vi "Obtain Broadcast Events.vi"(8 "error in (no error)":errorcluster, 10 "Create New?":bool) -> (0 "error out":errorcluster, 2 "FlexiFlowInterfaceCH2 Broadcast Events":T1)   [LabVIEW 2024, in "FlexiFlowInterfaceCH2.lvlib"]
doc: "This VI Obtains/Creates the Broadcast events that will be used for other modules to register to receive messages from the module that owns this VI.\n\n<b>NOTE</b>: The contents of this VI are automatically generated and modified by the <b>Tools > Delacor > DQMH</b> utilities. Consider using those utilities instead of making your own modifications to this VI.\n_____\nBased on Delacor QMH Project Template 3.1.0.34."
uses:
  FlexiFlowInterfaceCH2.lvlib
  Broadcast Events--cluster.ctl
  Did Init Argument--cluster.ctl
  Status Updated Argument--cluster.ctl
  Error Reported Argument--cluster.ctl
  Stop Argument--cluster.ctl
  Get Module Execution Status Argument--cluster.ctl
  Broadcast Device States Argument--cluster.ctl
  Modbus Flexi-Flow State--cluster.ctl
  <vilib>/Plasmionique/MB Master/MB_Master_TCP/MB_Master_TCP.lvclass
  Device Type--enum.ctl
  Modbus Flexi-Flow Controls--cluster.ctl
  Modbus Flexi-Flow API/Control Mode--enum.ctl
  Modbus Flexi-Flow API/Control Function Values--enum.ctl
  Modbus Flexi-Flow Measure State--cluster.ctl
  Broadcast State (Data Map) Argument--cluster.ctl
  Modbus Flexi-Flow API/Bronkhorst Flexi-Flow ModbusTCP API.lvlib
panel:
  # "NOTE: The contents of this VI are automatically generated and modified by the Tools > Delacor > DQMH utilities. Consider using those utilities instead of making your own modifications to this VI."
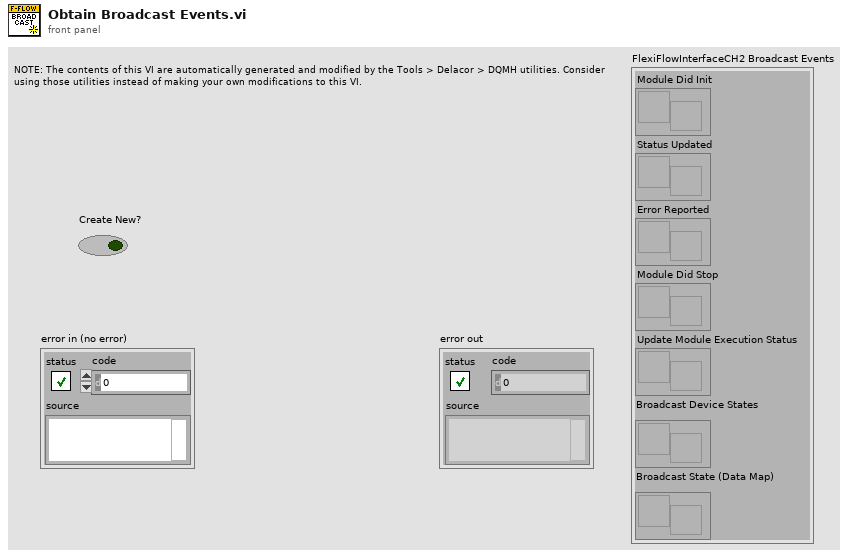
[diagram p1: front panel]
types:
  T1 = typedef "FlexiFlowInterfaceCH2.lvlib/Broadcast Events--cluster.ctl" = cluster{"Module Did Init":refnum<user-event>, "Status Updated":refnum<user-event>, "Error Reported":refnum<user-event>, "Module Did Stop":refnum<user-event>, "Update Module Execution Status":refnum<user-event>, "Broadcast Device States":refnum<user-event>, "Broadcast State (Data Map)":refnum<user-event>}
  T2 = typedef "FlexiFlowInterfaceCH2.lvlib/Broadcast State (Data Map) Argument--cluster.ctl" = cluster{"Data Table":map{string, dbl}}
  T3 = typedef "FlexiFlowInterfaceCH2.lvlib/Broadcast Device States Argument--cluster.ctl" = cluster{"Flexi-Flow Devices":T4[]}
  T4 = typedef "FlexiFlowInterfaceCH2.lvlib/Modbus Flexi-Flow State--cluster.ctl" = cluster{"Type":T5, "Label":string, "User Tag":string, "MB_TCP session":refnum<class "MB_Master_TCP.lvclass">, "Control State":T6, "Measurement State":T9}
  T5 = typedef "FlexiFlowInterfaceCH2.lvlib/Device Type--enum.ctl" = enum16{"Mass Flow Controller", "Mass Flow Meter"}
  T6 = typedef "FlexiFlowInterfaceCH2.lvlib/Modbus Flexi-Flow Controls--cluster.ctl" = cluster{"Control Mode":T7, "Function":T8, "FSetpoint":sgl, "Flow Capacity Unit":string, "Setpoint Slope":u16, "P1Setpoint":sgl, "P2Setpoint":sgl}
  T7 = typedef "Bronkhorst Flexi-Flow ModbusTCP API.lvlib/Control Mode--enum.ctl" = u16
  T8 = typedef "Bronkhorst Flexi-Flow ModbusTCP API.lvlib/Control Function Values--enum.ctl" = enum16{"Flow", "Upstream pressure", "Downstream pressure", "Flow with upstream pressure limit", "Flow with downstream pressure limit", "Upstream pressure with flow limit", "Downstream pressure with flow limit"}
  T9 = typedef "FlexiFlowInterfaceCH2.lvlib/Modbus Flexi-Flow Measure State--cluster.ctl" = cluster{"Fmeasure":dbl, "P1measure":sgl, "P2measure":sgl}
  T10 = typedef "FlexiFlowInterfaceCH2.lvlib/Get Module Execution Status Argument--cluster.ctl" = cluster{"Running?":bool}
  T11 = typedef "FlexiFlowInterfaceCH2.lvlib/Stop Argument--cluster.ctl" = cluster{"Origin":string, "Exit via Stop Module Req?":bool, "Wait for Module to stop?":bool}
  T12 = typedef "FlexiFlowInterfaceCH2.lvlib/Error Reported Argument--cluster.ctl" = cluster{"Error":errorcluster, "Additional Information":string, "Module Name":string}
  T13 = typedef "FlexiFlowInterfaceCH2.lvlib/Status Updated Argument--cluster.ctl" = cluster{"Status":string}
  T14 = typedef "FlexiFlowInterfaceCH2.lvlib/Did Init Argument--cluster.ctl" = cluster{"Init?":bool, "Info":string}
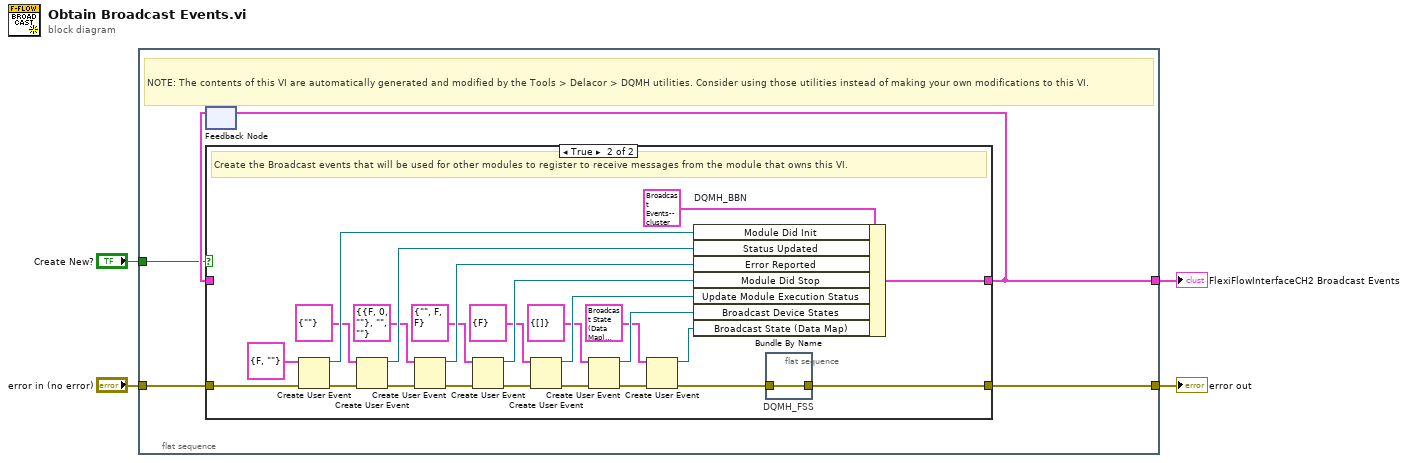
[diagram p0: block diagram]
diagram:
  n1 = flat-sequence {
    tunnel: [w9] -> w4
    tunnel: "error in (no error)" -> [w8]
    tunnel: [w6] -> w2
    tunnel: "Create New?" -> [w5]
    frame #0 {
      # "NOTE: The contents of this VI are automatically generated and modified by the Tools > Delacor > DQMH utilities. Consider using those utilities instead of making your own modifications to this VI."
      n2 = feedback #1() -> (w7:T1)  [unwired: 1 in]
      n3 = case shown="True" w5 {
        tunnel: [w10 w21] -> w9
        tunnel: w8 -> [w10 w36]
        tunnel: [w11 w33] -> w6
        tunnel: w7 -> [w11 _]
        frame False {
          # "Obtain the Broadcast events that were created in a previous call to this VI."
        }
        frame True {
          # "Create the Broadcast events that will be used for other modules to register to receive messages from the module that owns this VI."
          n4 = Create User Event(user event datatype=T14 {"Init?"=FALSE, "Info"=""} ("Did Init Argument"), error in=w36) -> (user event=w34:refnum<user-event>, error out=w31:errorcluster)
          n5 = Create User Event(user event datatype=T13 {"Status"=""} ("Status Updated Argument"), error in=w31) -> (user event=w28:refnum<user-event>, error out=w30:errorcluster)
          n6 = Create User Event(user event datatype=T12 {"Error"={"status"=FALSE, "code"=0, "source"=""}, "Additional Information"="", "Module Name"=""} ("Error Reported Argument"), error in=w30) -> (user event=w25:refnum<user-event>, error out=w27:errorcluster)
          n7 = Create User Event(user event datatype=T11 {"Origin"="", "Exit via Stop Module Req?"=FALSE, "Wait for Module to stop?"=FALSE} ("Stop Argument"), error in=w27) -> (user event=w23:refnum<user-event>, error out=w22:errorcluster)
          n8 = Create User Event(user event datatype=T10 {"Running?"=FALSE} ("Get Module Execution Status Argument"), error in=w22) -> (user event=w19:refnum<user-event>, error out=w20:errorcluster)
          n9 = Create User Event(user event datatype=T3 {"Flexi-Flow Devices"=[]} ("Broadcast Device States Argument"), error in=w20) -> (user event=w16:refnum<user-event>, error out=w17:errorcluster)
          n10 = Create User Event(user event datatype=T2 {"Data Table"={}} ("Broadcast State (Data Map) Argument"), error in=w17) -> (user event=w13:refnum<user-event>, error out=w14:errorcluster)
          n11 = Bundle By Name "DQMH_BBN"(cluster=T1 {"Module Did Init"=refnum, "Status Updated"=refnum, "Error Reported"=refnum, "Module Did Stop"=refnum, "Update Module Execution Status"=refnum, "Broadcast Device States"=refnum, "Broadcast State (Data Map)"=refnum} ("output cluster"), "Module Did Init"=w34, "Status Updated"=w28, "Error Reported"=w25, "Module Did Stop"=w23, "Update Module Execution Status"=w19, "Broadcast Device States"=w16, "Broadcast State (Data Map)"=w13) -> (w33:T1)
          n12 = flat-sequence "DQMH_FSS" {
            tunnel: w14 -> [w37]
            tunnel: [w37] -> w21
            frame #0 {
            }
          }
        }
      }
      n13 = feedback-in #1(w6) -> ()
    }
  }
  "FlexiFlowInterfaceCH2 Broadcast Events" <- w2
  "error out" <- w4
